vi "LVH5Rcreate (Object).vi"(6 "error in (no error)":errorcluster, 8 "Name":string, 9 "HDF5 Loc Ref":T1) -> (0 "error out":errorcluster, 2 "HDF5 Object Reference":T2, 3 "HDF5 Loc Ref out":T1)   [LabVIEW 2017]
doc: "Creates a reference."
uses:
  <vilib>/UPVI/lvhdf5/library.llb/HDF5 Ref.ctl
  <vilib>/UPVI/lvhdf5/reference.llb/H5R Object Ref.ctl
  <vilib>/UPVI/lvhdf5/dataspace.llb/H5S_class_t.ctl
  <vilib>/UPVI/lvhdf5/reference.llb/H5R_type_t.ctl
  <vilib>/UPVI/lvhdf5/h5helper.dll
panel:
  # "LVHDF5 Toolkit\nCopyright (c) 2005-2013 by Jason D. Sommerville\nCopyright (c) 2014 by UPVI, LLC.\n\nThis use and distribution of this file is governed by the terms found in \nLICENSE.txt distributed with this toolkit and installed at\n <user.lib>\\_lvhdf5\\LICENSE.txt"
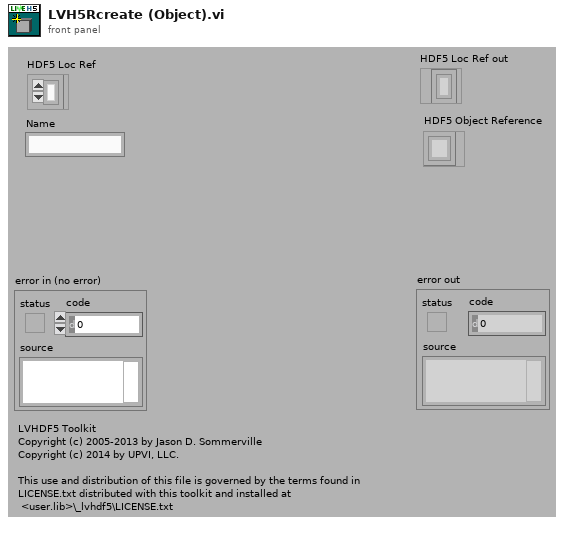
[diagram p1: front panel]
types:
  T1 = typedef "HDF5 Ref.ctl" = refnum<k1>
  T2 = typedef "H5R Object Ref.ctl" = refnum<k1>
  T3 = typedef "H5S_class_t.ctl" = i32
  T4 = typedef "H5R_type_t.ctl" = i32
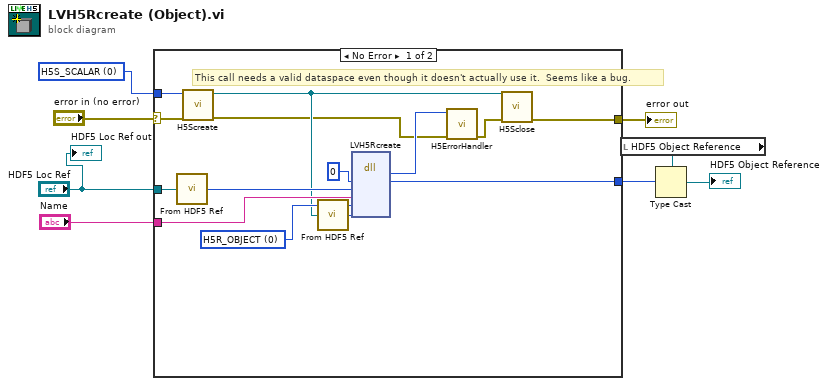
[diagram p0: block diagram]
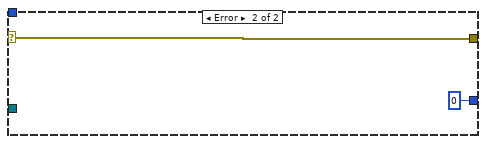
[diagram p2: hidden frame]
diagram:
  w1 = T3 0 items=["H5S_NONE"=-1, "H5S_SCALAR"=0, "H5S_SIMPLE"=1] ("Type")
  n1 = case shown="No Error" "error in (no error)" {
    selector: "error in (no error)" -> [w15 w24]
    tunnel: [w10 w24] -> w7
    tunnel: "HDF5 Loc Ref" -> [w21 _]
    tunnel: "Name" -> [w18 _]
    tunnel: [w16 0 ("pHandle")] -> w4
    tunnel: w1 -> [w14 _]
    frame No Error {
      w19 = T4 0 items=["H5R_BADTYPE"=-1, "H5R_OBJECT"=0, "H5R_DATASET_REGION"=1, "H5R_INTERNAL"=2] ("Reference Type")
      # "This call needs a valid dataspace even though it doesn't actually use it.  Seems like a bug."
      n2 = call <vilib>:"From HDF5 Ref.vi"("HDF5 Ref"=w21) -> ("I32"=w20:i32)
      n3 = call <vilib>:"H5Screate.vi"("error in (no error)"=w15, "Type"=w14) -> ("error out"=w9:errorcluster, "HDF5 Dataspace Ref"=w11:T1)  [unwired: 6 in]
      n4 = call <vilib>:"From HDF5 Ref.vi"("HDF5 Ref"=w11) -> ("I32"=w13:i32)
      n5 = dll-call lib="C:/Program Files/National Instruments/LabVIEW 2017/vi.lib/UPVI/lvhdf5/h5helper.dll" fn="LVH5Rcreate"("pHandle"=0, "loc_id"=w20, "name"=w18, "ref_type"=w19, "space_id"=w13) -> (w22:i32, "pHandle"=w16:i32)  [unwired: 7 in, 2 out]
      n6 = call <vilib>:"H5ErrorHandler.vi"("error in (no error)"=w9, "herr_t"=w22) -> ("error out"=w12:errorcluster)  [unwired: 3 in, 4 out]
      n7 = call <vilib>:"H5Sclose.vi"("error in (no error)"=w12, "HDF5 Dataspace Ref"=w11) -> ("error out"=w10:errorcluster)  [unwired: 7 in]
    }
    frame Error {
    }
  }
  "error out" <- w7
  n8 = local read "HDF5 Object Reference"() -> (w5:T2)
  n9 = Type Cast(type=w5, x=w4) -> (*(type *) &x=→"HDF5 Object Reference":T2)
  "HDF5 Loc Ref out" <- "HDF5 Loc Ref"
